vi "Error Handler.vi"(8 "error in (no error)":errorcluster, 9 "Message":string, 10 "Error Code":i32, 11 ".NET Refnum in":refnum<k24>) -> (0 "error out":errorcluster, 3 ".NET Refnum out":refnum<k24>)   [LabVIEW 2019, in "ESP301-Driver.lvlib"]
uses:
  ESP301-Driver.lvlib
  Newport.ESP301.CommandInterface
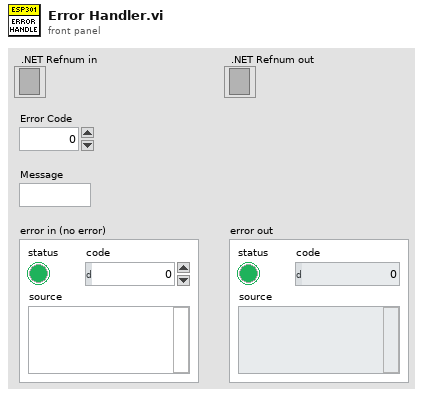
[diagram p1: front panel]
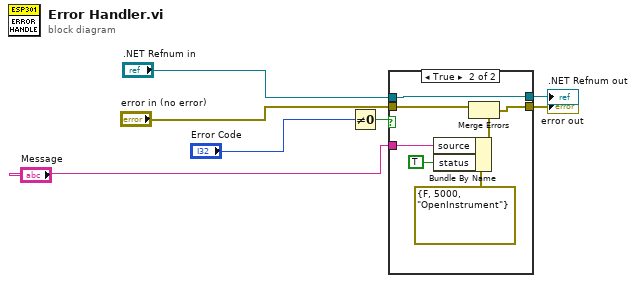
[diagram p0: block diagram]
diagram:
  n1 = Not Equal To 0?(x="Error Code") -> (x != 0?=w3:bool)
  n2 = case shown="True" w3 {
    tunnel: "error in (no error)" -> [w8 w16]
    tunnel: [w8 w15] -> w6
    tunnel: ".NET Refnum in" -> [w9 w11]
    tunnel: [w9 w11] -> w4
    tunnel: "Message" -> [_ w10]
    frame False {
    }
    frame True {
      n3 = Bundle By Name(cluster=errorcluster {"status"=FALSE, "code"=5000, "source"="OpenInstrument"} ("error in (no error)"), "source"=w10, "status"=TRUE) -> (w13:errorcluster)
      n4 = Merge Errors(w16, w13) -> (w15:errorcluster)
    }
  }
  ".NET Refnum out" <- w4
  "error out" <- w6
